vi "AnalogsRead.vi"(8 "Error in":errorcluster, 10 "Analog Input 2":tag[](array[tag]), 11 "Analog Input 1":tag[](array[tag])) -> (0 "Error out":errorcluster, 2 "Voltage Output 2":dbl, 3 "Voltage Output 1":dbl)   [LabVIEW 2021]
uses:
  <vilib>/Utility/error.llb/Error Cluster From Error Code.vi
  <vilib>/myRIO/Common/Instrument Driver Framework/myRIO v1.0/AI/vis/myRIO v1.0 Read AI.vi
  <vilib>/myRIO/Instrument Drivers/Onboard IO/AI/AI.lvlib
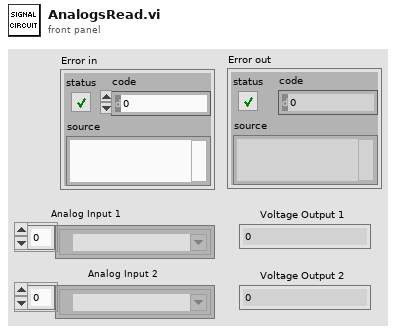
[diagram p1: front panel]
types:
  T1 = typedef "AI.lvlib/AI Reference.ctl" = cluster{"myRIO Reference":T2, "AI Channels List":T6, "AI Scaling Constants List":T8}
  T2 = typedef "myRIO Generic Hardware Reference.ctl" = cluster{"myRIO Model":T3, "myRIO Hardware Reference":T4}
  T3 = typedef "Hardware Version Enum.ctl" = enum16{"Unknown", "myRIO-1900", "myRIO-1950", "roboRIO", "NI ELVIS RIO CM", "ELVIS III"}
  T4 = typedef "myRIO v1.0 Reference.ctl" = cluster{"Generic FPGA Reference":T5, "Allow multiple opens":bool}
  T5 = typedef "Generic FPGA Reference.ctl" = refnum<k20>
  T6 = typedef "AI Channels List.ctl" = T7[]
  T7 = typedef "AI Channels Enum.ctl" = enum16{"Not Connected", "AudioIn/Left", "AudioIn/Right", "C/AI0", "C/AI1", "A/AI0", "A/AI1", "A/AI2", "A/AI3", "A/AI4", "A/AI5", "A/AI6", "A/AI7", "B/AI0", "B/AI1", "B/AI2", "B/AI3", "B/AI4", "B/AI5", "B/AI6", "B/AI7", "AI/AI0", "AI/AI1", "AI/AI2", "AI/AI3", "A/AI0 (DIFF)", "A/AI1 (DIFF)", "A/AI2 (DIFF)", "A/AI3 (DIFF)", "B/AI0 (DIFF)", "B/AI1 (DIFF)", "B/AI2 (DIFF)", "B/AI3 (DIFF)"}
  T8 = typedef "Analog Scaling Constants List.ctl" = T9[]
  T9 = typedef "Analog Scaling Constants.ctl" = cluster{"LSB Weight (Volts)":dbl, "Offset (Volts)":dbl, "Signed?":bool}
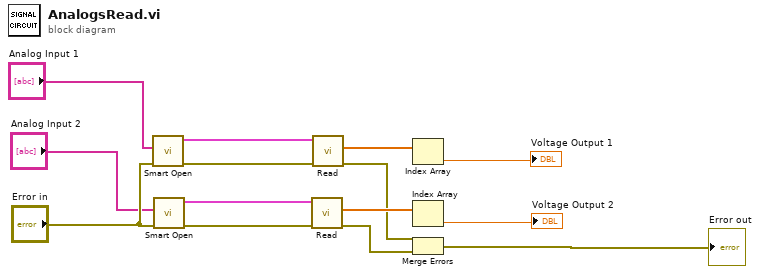
[diagram p0: block diagram]
diagram:
  n1 = call <vilib>:"Smart Open.vi"("error in (no error)"="Error in", "Channel Names"="Analog Input 1") -> ("error out"=w13:errorcluster, "AI Ref Out"=w12:T1)  [unwired: 8 in]
  n2 = call <vilib>:"Smart Open.vi"("error in (no error)"="Error in", "Channel Names"="Analog Input 2") -> ("error out"=w9:errorcluster, "AI Ref Out"=w8:T1)  [unwired: 8 in]
  n3 = call <vilib>:"Read.vi"("error in (no error)"=w9, "AI Ref In"=w8) -> ("error out"=w4:errorcluster, "Values"=w5:dbl[])  [unwired: 7 in, 1 out]
  n4 = call <vilib>:"Read.vi"("error in (no error)"=w13, "AI Ref In"=w12) -> ("error out"=w3:errorcluster, "Values"=w6:dbl[])  [unwired: 7 in, 1 out]
  n5 = Index Array(array=w6) -> (element=→"Voltage Output 1":dbl)  [unwired: 1 in]
  n6 = Index Array(array=w5) -> (element=→"Voltage Output 2":dbl)  [unwired: 1 in]
  n7 = Merge Errors(w3, w4) -> (→"Error out":errorcluster)
